vi "Calibrate_Axis.vi"() -> ()   [LabVIEW 2015]
uses:
  Camera Server/Camera enum/Camera enum.ctl
  Anemometry Sub Vis/Gen Trav/Traverse_cluster.ctl
  Anemometry Sub Vis/Gen Trav/Spacing.ctl
  Anemometry Sub Vis/Controls/Multi_run_mode.ctl
  Image acquisition and processing/Feature detection/Typedefs/Top level controls.ctl
  Image acquisition and processing/Feature detection/Typedefs/Theta range.ctl
  Image acquisition and processing/Feature detection/Typedefs/Txy range.ctl
  Image acquisition and processing/Feature detection/Typedefs/ROI bounds.ctl
  Anemometry Sub Vis/Controls/Tunnel_Coordinates.ctl
  Anemometry Sub Vis/Globals/Constants_global.vi
  Anemometry Sub Vis/Globals/Meas_global.vi
panel:
  in  "Traverse Name":string
  in  "Camera":T1="Pencilcam"
  in  "Axis to Calibrate":enum16{"X Axis", "Y Axis"}(ring)
  in  "Min Position":dbl
  in  "Max Position":dbl
  in  "Datum Position":sgl[](array[numeric])=[0.0, 0.0, 0.0] format="%#.2f"
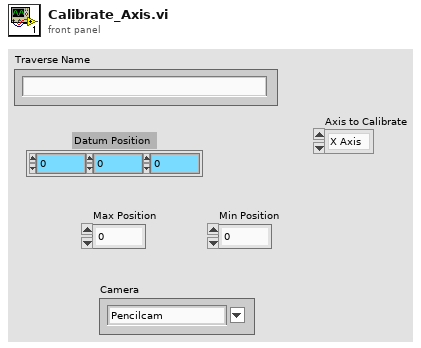
[diagram p1: front panel]
types:
  T1 = typedef "Camera enum.ctl" = string
  T2 = typedef "Traverse_cluster.ctl" = cluster{"Start X":sgl, "Start Y":sgl, "Start Z":sgl, "End X":sgl, "End Y":sgl, "End Z":sgl, "No. of pts.":i32, "Spacing":T3, "Filename":path, "Tunnel Speed":dbl, "Averaging time (min)":dbl, "Extra Commands":string, "Carrier_1 Q (l/min)":dbl, "Carrier_2 Q (l/min)":dbl, "Trace Gas Concentration (%)":dbl, "Specific Arguments":string, "Comments":string, "Row No":i32, "Row Type Selector":T4, "Completion time":string, "Row Duration (mins)":dbl, "No. of Valid pts.":i32, "Meas Setup File":string}
  T3 = typedef "Spacing.ctl" = enum16{"Linear", "Log", "Gauss", "Specified", "N/A"}
  T4 = typedef "Multi_run_mode.ctl" = enum16{"Move Traverse Only", "Set Tunnel Speed Only", "Set Source Only", "Set Measurement Conditions", "Single Measurement", "Vertical Profile", "Lateral Profile", "Longitudinal Profile", "Explore Volume", "Multi-Axis Profile", "Auto Calibrate", "Meas Fast FID Bkgnd", "Check Beam Power", "Scanning Valve Measurement", "Run VI Named:", "Set ADAM Ch", "Wait (minutes)", "Send Message", "Synchronize With:", "Fall Back to this Row", "Turn Off Row Repeating", "Blank Row", "Traverse 3D Volume"}
  T5 = typedef "ROI bounds.ctl" = cluster{"Xmax":i32, "Ymax":i32, "Xmin":i32, "Ymin":i32}
  T6 = typedef "Txy range.ctl" = cluster{"Tx max (pix)":i32, "Tx min (pix)":i32, "Ty max (pix)":i32, "Ty min (pix)":i32}
  T7 = typedef "Theta range.ctl" = cluster{"theta max (deg)":dbl, "theta min (deg)":dbl}
  T8 = typedef "Top level controls.ctl" = cluster{"Auto ROI (for rot.)":bool, "Apply scaling":bool, "Apply rotation":bool, "Apply Tx":bool, "Apply Ty":bool, "Keep proc. img":bool}
  T9 = enum16{"Load Command File", "Save Command File", "Check Multi Run Prog", "Check Multi Run Prog With Live Moves", "Run Multi Run Prog"}
  T10 = typedef "Tunnel_Coordinates.ctl" = enum16{"Work in Tunnel Coordinates", "Work in Model Coordinates"}
  T11 = enum16{"Load Command File", "Save Command File", "Check Multi Run Prog", "Check Multi Run Prog With Live Moves", "Run Multi Run Prog"}[]
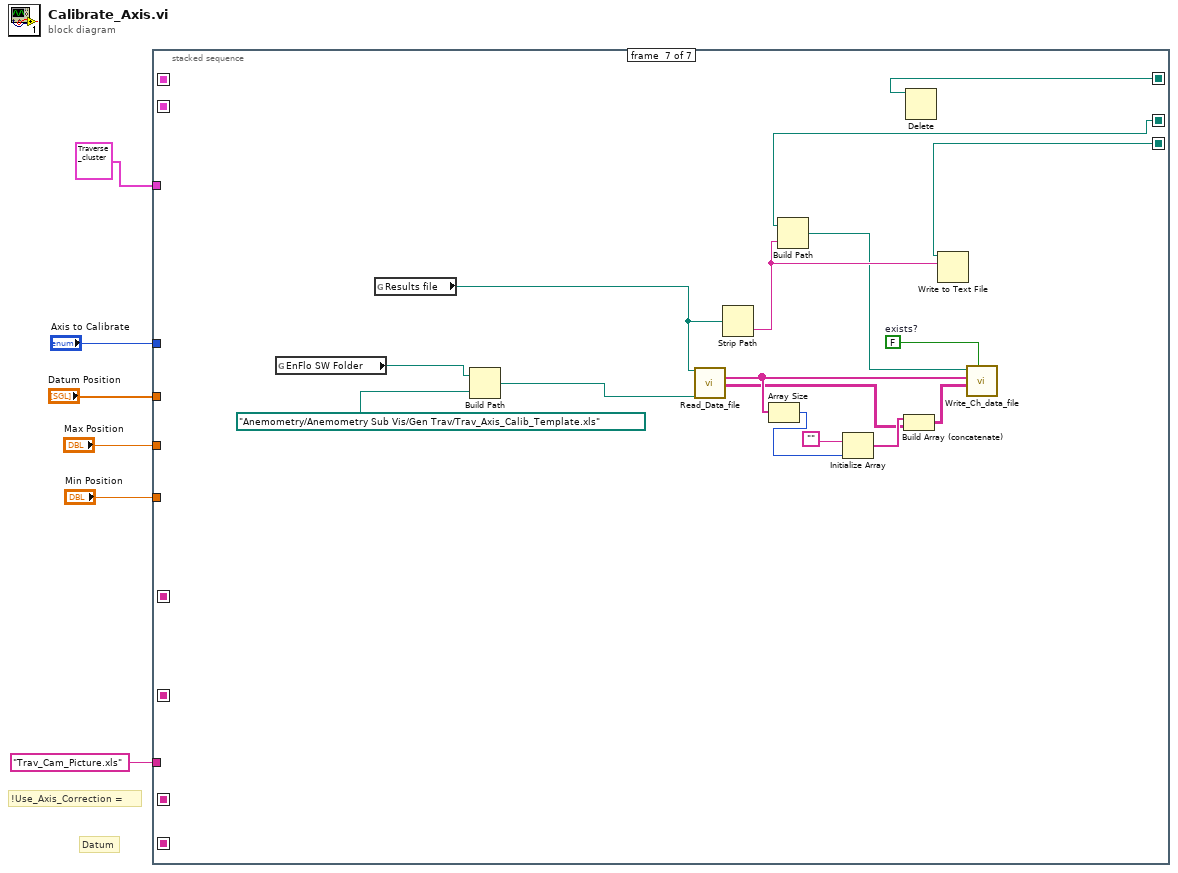
[diagram p0: block diagram]
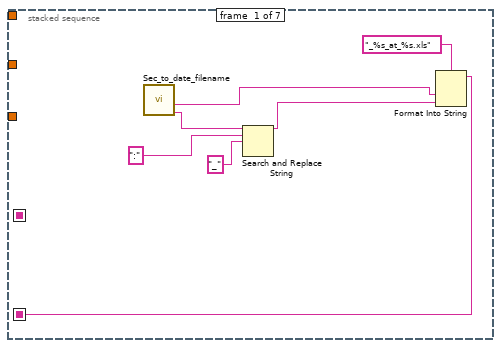
[diagram p2: hidden frame]
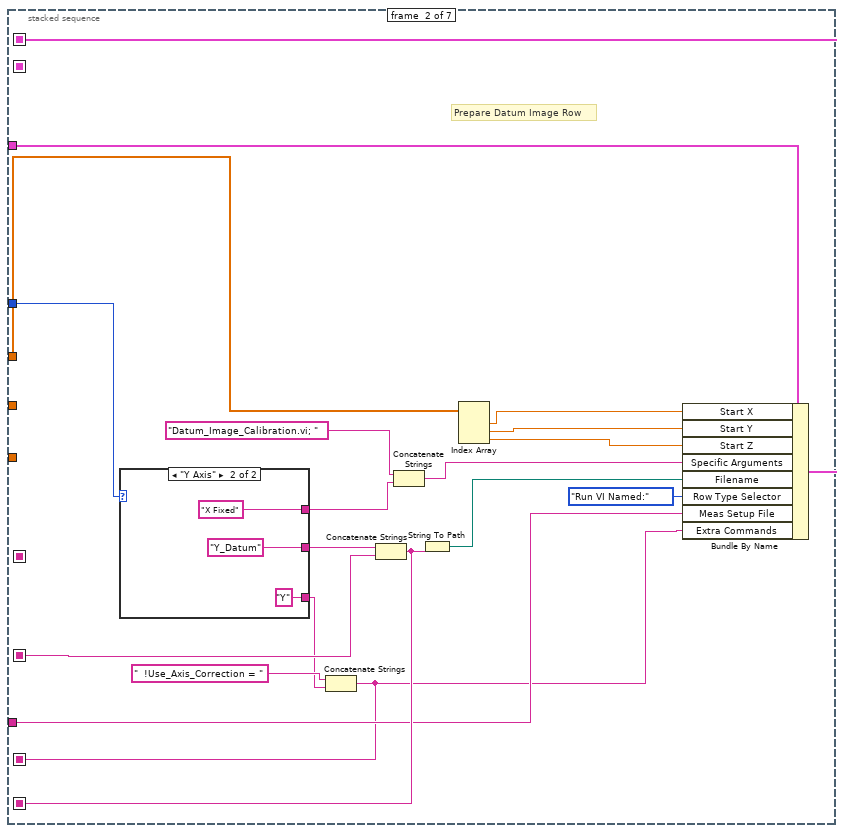
[diagram p3: hidden frame]
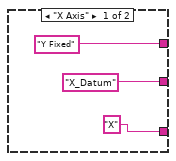
[diagram p4: hidden frame]
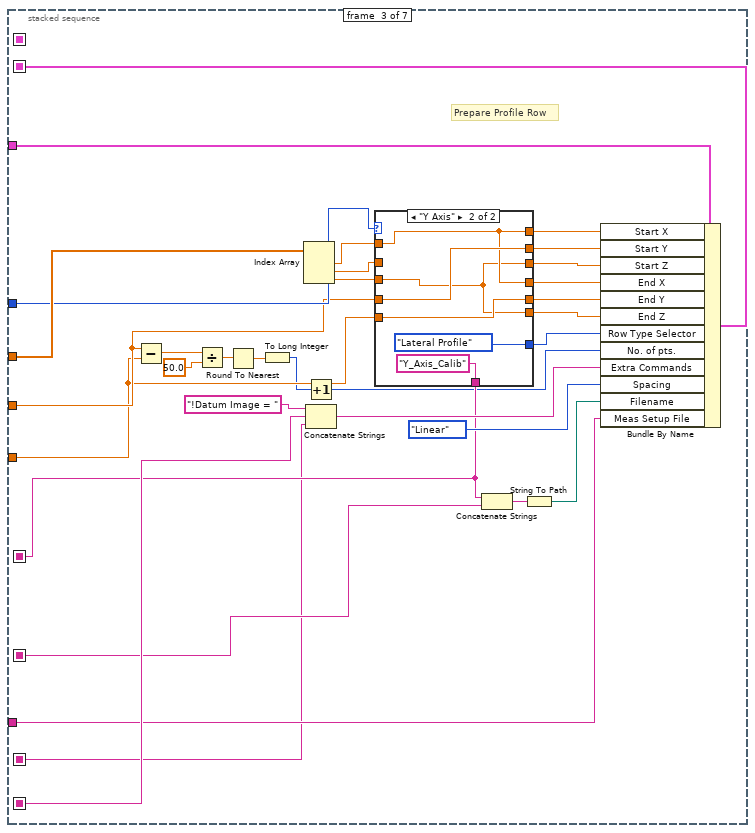
[diagram p5: hidden frame]
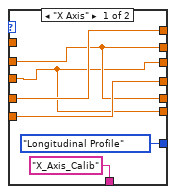
[diagram p6: hidden frame]
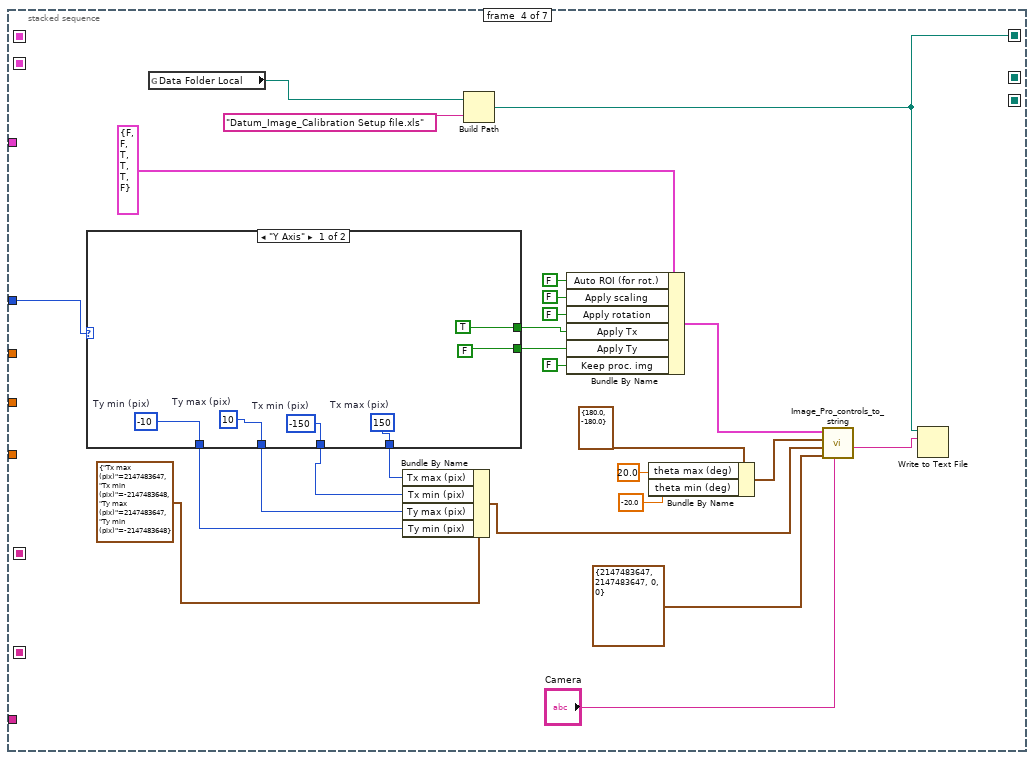
[diagram p7: hidden frame]
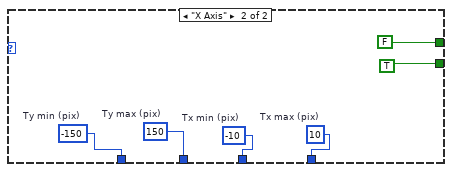
[diagram p8: hidden frame]
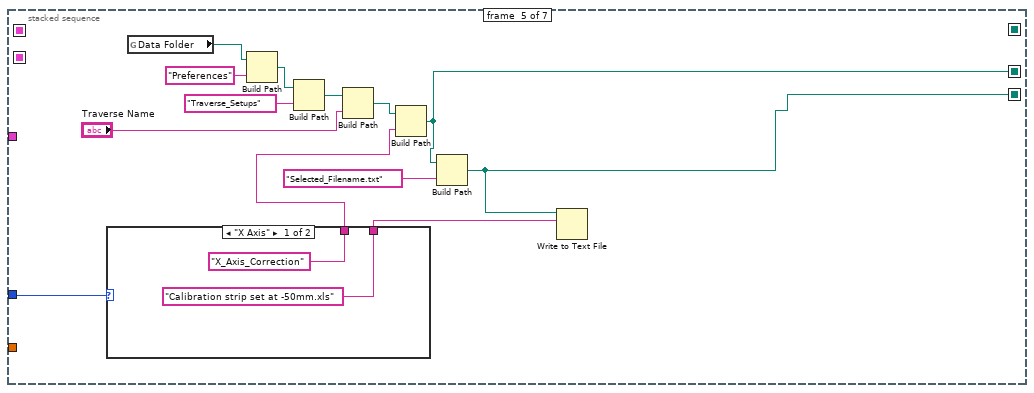
[diagram p9: hidden frame]
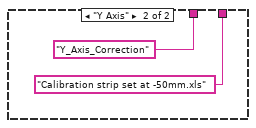
[diagram p10: hidden frame]
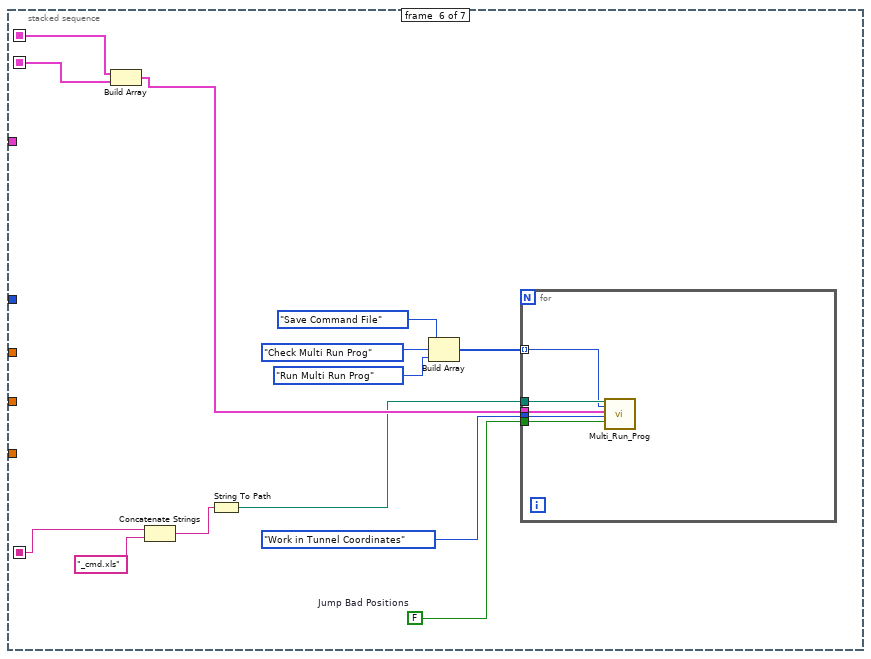
[diagram p11: hidden frame]
diagram:
  # "!Use_Axis_Correction ="
  # "Datum"
  n1 = stacked-sequence {
    seq-local: [_ w28 _ _ _ _ _] -> [_ _ _ _ _ w149 _]
    seq-local: [_ _ w48 _ _ _ _] -> [_ _ _ _ _ w148 _]
    seq-local: [w7 _ _ _ _ _ _] -> [_ w22 w46 _ _ _ _]
    seq-local: [_ w20 _ _ _ _ _] -> [_ _ w57 _ _ _ _]
    seq-local: [_ _ w41 _ _ _ _] -> [_ _ _ _ _ w146 _]
    seq-local: [_ _ _ w83 _ _ _] -> [_ _ _ _ _ _ w170]
    seq-local: [_ w14 _ _ _ _ _] -> [_ _ w39 _ _ _ _]
    seq-local: [_ _ _ _ w122 _ _] -> [_ _ _ _ _ _ w165]
    seq-local: [_ _ _ _ w121 _ _] -> [_ _ _ _ _ _ w164]
    tunnel: "Datum Position" -> [_ w32 w70 _ _ _ _]
    tunnel: "Axis to Calibrate" -> [_ w27 w69 w105 w125 _ _]
    tunnel: "Max Position" -> [_ _ w56 _ _ _ _]
    tunnel: "Min Position" -> [_ _ w55 _ _ _ _]
    tunnel: "Trav_Cam_Picture.xls" ("Meas Setup File") -> [_ w19 w43 _ _ _ _]
    tunnel: T2 {"Start X"=2010.0, "Start Y"=1100.0, "Start Z"=50.0, "End X"=2010.0, "End Y"=-1300.0, "End Z"=50.0, "No. of pts."=49, "Spacing"=enum."Linear", "Filename"=path "E:/Enflo_Data_Local/2016/EnFlo_Tunnel/Paul_Hayden/Results/Res_04-2016/Y_Axis_Calibration_Y+100.xls", "Tunnel Speed"=0.0, "Averaging time (min)"=0.05, "Extra Commands"="!Datum Image = 50mm_Y_Strip.xls", "Carrier_1 Q (l/min)"=0.0, "Carrier_2 Q (l/min)"=0.0, "Trace Gas Concentration (%)"=0.0, "Specific Arguments"="Y= ;1100 ; 1050 ; 1000 ; 950 ; 900 ; 850 ; 800 ; 750 ; 700 ; 650 ; 600 ; 550 ; 500 ; 450 ; 400 ; 350 ; 300 ; 250 ; 200 ; 150 ; 100 ; 50 ; 0 ; -50 ; -100 ; -150 ; -200 ; -250 ; -300 ; -350 ; -400 ; -450 ; -500 ; -550 ; -600 ; -650 ; -700 ; -750 ; -800 ; -850 ; -900 ; -950 ; -1000 ; -1050 ; -1100 ; -1150 ; -1200 ; -1250 ; -1300 ; ", "Comments"="", "Row No"=1, "Row Type Selector"=enum."Lateral Profile", "Completion time"="10:16  04-04-2016", "Row Duration (mins)"=10.616666666666667, "No. of Valid pts."=49, "Meas Setup File"="Trav_Cam_Picture.xls"} ("Traverse line") -> [_ w17 w42 _ _ _ _]
    frame #0 {
      n2 = call "Sec_to_date_filename.vi"() -> ("Day"=w11:string, "Time"=w8:string)  [unwired: 1 in, 2 out]
      n3 = Search and Replace String(input string=w8, search string=":", replace string="_" ("replace string (\"\")")) -> (result string=w12:string)  [unwired: 5 in, 3 out]
      n4 = Format Into String(format string="_%s_at_%s.xls", w11, w12) -> (resulting string=w7:string)  [unwired: 2 in, 1 out]
    }
    frame #1 {
      # "Prepare Datum Image Row"
      n5 = case shown="\"Y Axis\"" w27 {
        tunnel: ["Y Fixed" "X Fixed"] -> w25
        tunnel: ["X_Datum" ("format string") "Y_Datum" ("format string")] -> w23
        tunnel: ["X" ("format string") "Y" ("format string")] -> w15
        frame "X Axis" {
        }
        frame "Y Axis" {
        }
      }
      n6 = Concatenate Strings("  !Use_Axis_Correction = ", w15) -> (w14:string)
      n7 = Concatenate Strings(w23, w22) -> (w20:string)
      n8 = Concatenate Strings("Datum_Image_Calibration.vi; " ("Specific Arguments"), w25) -> (w24:string)
      n9 = String To Path(string=w20) -> (path=w21:path)
      n10 = Index Array(array=w32) -> (element #1=w31:sgl, element #2=w30:sgl, element #3=w29:sgl)  [unwired: 3 in]
      n11 = Bundle By Name(cluster=w17, "Start X"=w31, "Start Y"=w30, "Start Z"=w29, "Specific Arguments"=w24, "Filename"=w21, "Row Type Selector"=Multi_run_mode."Run VI Named:", "Meas Setup File"=w19, "Extra Commands"=w14) -> (w28:T2)
    }
    frame #2 {
      # "Prepare Profile Row"
      n12 = Subtract(x=w56, y=w55) -> (x-y=w54:dbl)
      n13 = Divide(x=w54, y=50.0) -> (x/y=w52:dbl)
      n14 = Round To Nearest(number=w52) -> (nearest integer value=w51:dbl)
      n15 = To Long Integer(number=w51) -> (32bit integer=w50:i32)
      n16 = Index Array(array=w70) -> (element #1=w66:sgl, element #2=w60:sgl, element #3=w63:sgl)  [unwired: 3 in]
      n17 = Increment(x=w50) -> (x+1=w40:i32)
      n18 = Concatenate Strings("!Datum Image = " ("Extra Commands"), w57, w39) -> (w49:string)
      n19 = case shown="\"Y Axis\"" w69 {
        tunnel: [w74 w82] -> w68
        tunnel: w56 -> [w76 w82]
        tunnel: w55 -> [w75 w81]
        tunnel: [w74 w81] -> w67
        tunnel: w66 -> [_ w80]
        tunnel: [w76 w80] -> w65
        tunnel: [w73 w79] -> w64
        tunnel: w63 -> [w73 w79]
        tunnel: [w75 w80] -> w62
        tunnel: [w73 w79] -> w61
        tunnel: w60 -> [w74 _]
        tunnel: [Multi_run_mode."Longitudinal Profile" ("Row Type Selector") Multi_run_mode."Lateral Profile" ("Row Type Selector")] -> w59
        tunnel: ["X_Axis_Calib" ("format string") "Y_Axis_Calib" ("format string")] -> w41
        frame "X Axis" {
        }
        frame "Y Axis" {
        }
      }
      n20 = Concatenate Strings(w41, w46) -> (w45:string)
      n21 = String To Path(string=w45) -> (path=w44:path)
      n22 = Bundle By Name(cluster=w42, "Start X"=w65, "Start Y"=w68, "Start Z"=w64, "End X"=w62, "End Y"=w67, "End Z"=w61, "Row Type Selector"=w59, "No. of pts."=w40, "Extra Commands"=w49, "Spacing"=Spacing."Linear", "Filename"=w44, "Meas Setup File"=w43) -> (w48:T2)
    }
    frame #3 {
      n23 = case shown="\"Y Axis\"" w105 {
        tunnel: [FALSE ("Apply Ty") TRUE ("Apply Ty")] -> w99
        tunnel: [TRUE ("Apply Tx") FALSE ("Apply Tx")] -> w98
        tunnel: [w111 w117] -> w91
        tunnel: [w110 w116] -> w90
        tunnel: [w109 w115] -> w89
        tunnel: [w108 w114] -> w88
        frame "Y Axis" {
          w110 = -150  # Tx min (pix)
          w109 = 10  # Ty max (pix)
          w108 = -10  # Ty min (pix)
          w111 = 150  # Tx max (pix)
        }
        frame "X Axis" {
          w116 = -10  # Tx min (pix)
          w115 = 150  # Ty max (pix)
          w114 = -150  # Ty min (pix)
          w117 = 10  # Tx max (pix)
        }
      }
      n24 = global read "Constants_global.vi" "Data Folder Local"() -> (w106:path)
      n25 = Bundle By Name(cluster=T6 {"Tx max (pix)"=2147483647, "Tx min (pix)"=-2147483648, "Ty max (pix)"=2147483647, "Ty min (pix)"=-2147483648} ("Txy range (pixels)"), "Tx max (pix)"=w91, "Tx min (pix)"=w90, "Ty max (pix)"=w89, "Ty min (pix)"=w88) -> (w87:T6)
      n26 = Build Path(base path=w106, name or relative path="Datum_Image_Calibration Setup file.xls") -> (appended path=w83:path)
      n27 = Bundle By Name(cluster=T8 {"Auto ROI (for rot.)"=FALSE, "Apply scaling"=FALSE, "Apply rotation"=TRUE, "Apply Tx"=TRUE, "Apply Ty"=TRUE, "Keep proc. img"=FALSE} ("Controls"), "Auto ROI (for rot.)"=FALSE, "Apply scaling"=FALSE, "Apply rotation"=FALSE, "Apply Tx"=w98, "Apply Ty"=w99, "Keep proc. img"=FALSE) -> (w97:T8)
      n28 = Bundle By Name(cluster=T7 {"theta max (deg)"=180.0, "theta min (deg)"=-180.0} ("Theta range (deg)"), "theta max (deg)"=20.0, "theta min (deg)"=-20.0) -> (w95:T7)
      n29 = call "Image_Pro_controls_to_string.vi"("Camera"="Camera", "ROI to crop (pixels)"=T5 {"Xmax"=2147483647, "Ymax"=2147483647, "Xmin"=0, "Ymin"=0}, "Txy range (pixels)"=w87, "Theta range (deg)"=w95, "Controls"=w97) -> ("Setup String"=w84:string)  [unwired: 6 in]
      n30 = Write to Text File(file (use dialog)=w83, text=w84) -> ()  [unwired: 2 in, 3 out]
    }
    frame #4 {
      n31 = case shown="\"X Axis\"" w125 {
        tunnel: ["Calibration strip set at -50mm.xls" "Calibration strip set at -50mm.xls"] -> w120
        tunnel: ["X_Axis_Correction" ("name or relative path") "Y_Axis_Correction" ("name or relative path")] -> w123
        frame "X Axis" {
        }
        frame "Y Axis" {
        }
      }
      n32 = global read "Constants_global.vi" "Data Folder"() -> (w129:path)
      n33 = Build Path(base path=w129, name or relative path="Preferences") -> (appended path=w131:path)
      n34 = Build Path(base path=w131, name or relative path="Traverse_Setups") -> (appended path=w132:path)
      n35 = Build Path(base path=w132, name or relative path="Traverse Name") -> (appended path=w124:path)
      n36 = Build Path(base path=w124, name or relative path=w123) -> (appended path=w122:path)
      n37 = Build Path(base path=w122, name or relative path="Selected_Filename.txt" ("Substring")) -> (appended path=w121:path)
      n38 = Write to Text File(file (use dialog)=w121, text=w120) -> ()  [unwired: 2 in, 3 out]
    }
    frame #5 {
      w141 = FALSE  # Jump Bad Positions
      n39 = Build Array(w149, w148) -> (w147:T2[])
      n40 = Concatenate Strings(w146, "_cmd.xls" ("string")) -> (w143:string)
      n41 = String To Path(string=w143) -> (path=w144:path)
      n42 = Build Array(T9."Save Command File" ("Mode"), T9."Check Multi Run Prog" ("Mode"), T9."Run Multi Run Prog" ("Mode")) -> (w137:T11)
      n43 = for {
        tunnel: w147 -> [w154]
        tunnel: w144 -> [w153]
        tunnel: Tunnel_Coordinates."Work in Tunnel Coordinates" ("Work in Tunnel Coordinates?") -> [w152]
        tunnel: w141 -> [w151]
        tunnel: w137 -> [w150] mode=indexing
        n44 = call "Multi_Run_Prog.vi"("Command filename"=w153, "Mode"=w150, "Table"=w154, "Work in Tunnel Coordinates?"=w152, "Jump Bad Positions"=w151) -> ()  [unwired: 15 in]
      }
    }
    frame #6 {
      w161 = FALSE  # exists?
      n45 = global read "Constants_global.vi" "EnFlo SW Folder"() -> (w169:path)
      n46 = global read "Meas_global.vi" "Results file"() -> (w166:path)
      n47 = Build Path(base path=w169, name or relative path=path "Anemometry/Anemometry Sub Vis/Gen Trav/Trav_Axis_Calib_Template.xls") -> (appended path=w167:path)
      n48 = call "Read_Data_file.vi"("Results file"=w166, "Template File"=w167) -> ("Ch names Out"=w160:string[], "Channel Values Out"=w156:string[][])  [unwired: 3 in, 13 out]
      n49 = Strip Path(path=w166) -> (name=w163:string)  [unwired: 1 out]
      n50 = Array Size(array=w160) -> (size(s)=w159:i32)
      n51 = Build Path(base path=w165, name or relative path=w163) -> (appended path=w162:path)
      n52 = Initialize Array("", w159) -> (w157:string[])
      n53 = Build Array (concatenate)(w157, w156) -> (w155:string[][])
      n54 = Delete(path (use dialog)=w170) -> ()  [unwired: 4 in, 3 out]
      n55 = Write to Text File(file (use dialog)=w164, text=w163) -> ()  [unwired: 2 in, 3 out]
      n56 = call "Write_Ch_data_file.vi"("exists?"=w161, "Channel Values"=w155, "Channel names"=w160, "Filename"=w162) -> ()  [unwired: 3 in, 5 out]
    }
  }
